vi "serial_read_write.vi"(10 "Enable Delayline":bool, 11 "VISA Refnum in":refnum<visa-resource-name>="COM4") -> ()   [LabVIEW 2024]
uses:
  <vilib>/Instr/_visa.llb/VISA Configure Serial Port (Instr).vi
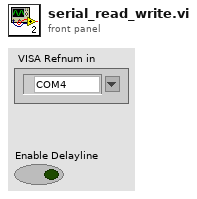
[diagram p1: front panel]
types:
  T1 = cluster{"baud rate":u32, "data bits":u16, "parity":dbl, "stop bits":u16, "flow control":u16}
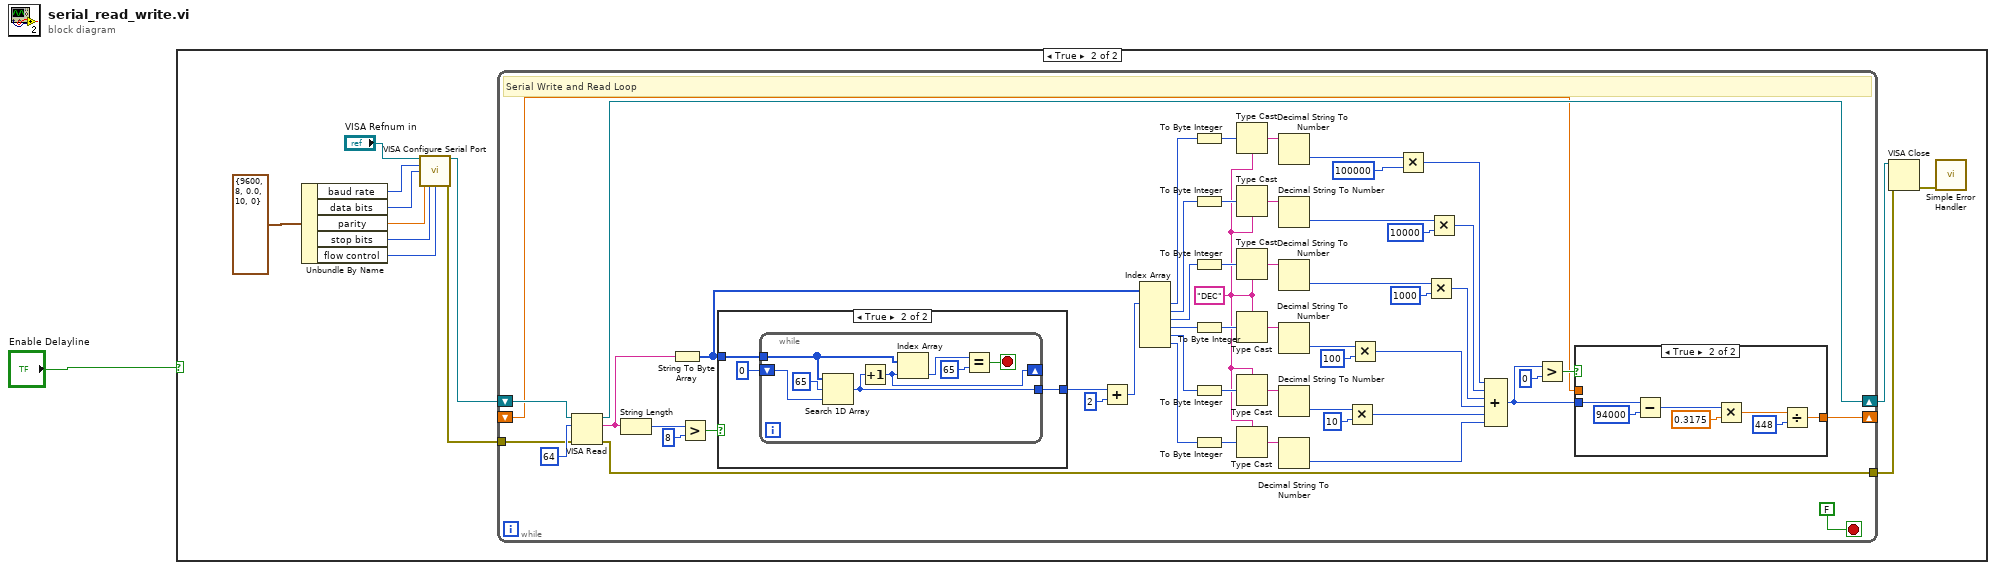
[diagram p0: block diagram]
diagram:
  n1 = case shown="True" "Enable Delayline" {
    frame False {
    }
    frame True {
      n2 = Unbundle By Name(T1 {"baud rate"=9600, "data bits"=8, "parity"=0.0, "stop bits"=10, "flow control"=0} ("Serial Settings")) -> ("baud rate"=w9:u32, "data bits"=w10:u16, "parity"=w11:dbl, "stop bits"=w12:u16, "flow control"=w4:u16)
      n3 = call-poly "VISA Configure Serial Port"("VISA resource name"="VISA Refnum in", "baud rate (9600)"=w9, "data bits (8)"=w10, "parity (0:none)"=w11, "stop bits (10: 1 bit)"=w12, "flow control (0:none)"=w4) -> ("VISA resource name out"=w2:refnum<visa-resource-name>, "error out"=w3:errorcluster)  [unwired: 4 in, 4 out]
      n4 = while {
        shift-right: [w66] -> w5
        shift-left: w2 -> [w32]
        tunnel: [w65] -> w6
        tunnel: w3 -> [w33]
        shift-right: [w15] -> _
        shift-left: _ -> [w14]
        stop <- FALSE stop-if-true
        w25 = "DEC"
        # "Serial Write and Read Loop"
        n5 = VISA Read(VISA resource name=w32, byte count=u32 64 ("Read Count"), error in (no error)=w33) -> (VISA resource name out=w66:refnum<visa-resource-name>, read buffer=w37:string, error out=w65:errorcluster)  [unwired: 1 out]
        n6 = String Length(string=w37) -> (length=w36:i32)
        n7 = String To Byte Array(string=w37) -> (unsigned byte array=w62:u8[])
        n8 = Greater?(x=w36, y=8) -> (0:w34:bool)
        n9 = case shown="True" w34 {
          tunnel: w62 -> [_ w78]
          tunnel: [_ w77] -> w60
          frame False {
          }
          frame True {
            n10 = while {
              shift-right: [w80] -> _
              shift-left: 0 -> [w82]
              tunnel: w78 -> [w83]
              tunnel: [w79] -> w77
              stop <- w81 stop-if-true
              n11 = Search 1D Array(1D array=w83, element=65, start index (0)=w82) -> (index of element=w79:i32)
              n12 = Increment(x=w79) -> (x+1=w80:i32)
              n13 = Index Array(array=w83, index=w80) -> (element=w85:u8)
              n14 = Equal?(x=w85, y=65) -> (x = y?=w81:bool)
            }
          }
        }
        n15 = Add(x=w60, y=2) -> (x+y=w61:i32)
        n16 = Index Array(array=w62, index #1=w61) -> (element #1=w59:u8, element #2=w58:u8, element #3=w57:u8, element #4=w56:u8, element #5=w55:u8, element #6=w27:u8)  [unwired: 5 in]
        n17 = To Byte Integer(number=w59) -> (8bit integer=w31:i8)
        n18 = To Byte Integer(number=w58) -> (8bit integer=w54:i8)
        n19 = To Byte Integer(number=w57) -> (8bit integer=w53:i8)
        n20 = To Byte Integer(number=w56) -> (8bit integer=w52:i8)
        n21 = To Byte Integer(number=w55) -> (8bit integer=w51:i8)
        n22 = To Byte Integer(number=w27) -> (8bit integer=w26:i8)
        n23 = Type Cast(type=w25, x=w31) -> (*(type *) &x=w30:string)
        n24 = Type Cast(type=w25, x=w54) -> (*(type *) &x=w50:string)
        n25 = Type Cast(type=w25, x=w53) -> (*(type *) &x=w49:string)
        n26 = Type Cast(type=w25, x=w52) -> (*(type *) &x=w48:string)
        n27 = Type Cast(type=w25, x=w51) -> (*(type *) &x=w47:string)
        n28 = Type Cast(type=w25, x=w26) -> (*(type *) &x=w20:string)
        n29 = Decimal String To Number(string=w30) -> (number=w23:i32)  [unwired: 2 in, 1 out]
        n30 = Decimal String To Number(string=w50) -> (number=w45:i32)  [unwired: 2 in, 1 out]
        n31 = Decimal String To Number(string=w49) -> (number=w44:i32)  [unwired: 2 in, 1 out]
        n32 = Decimal String To Number(string=w48) -> (number=w42:i32)  [unwired: 2 in, 1 out]
        n33 = Decimal String To Number(string=w47) -> (number=w22:i32)  [unwired: 2 in, 1 out]
        n34 = Decimal String To Number(string=w20) -> (number=w19:i32)  [unwired: 2 in, 1 out]
        n35 = Multiply(x=w22, y=10) -> (x*y=w24:i32)
        n36 = Multiply(x=w42, y=100) -> (x*y=w38:i32)
        n37 = Multiply(x=w23, y=100000) -> (x*y=w28:i32)
        n38 = Multiply(x=w44, y=1000) -> (x*y=w39:i32)
        n39 = Multiply(x=w45, y=10000) -> (x*y=w40:i32)
        n40 = Compound Arithmetic op=ADD(w28, w40, w39, w38, w24, w19) -> (w16:i32)
        n41 = Greater?(x=w16, y=0) -> (0:w17:bool)
        n42 = case shown="True" w17 {
          tunnel: [w68 w69] -> w15
          tunnel: w16 -> [_ w75]
          tunnel: w14 -> [w68 _]
          frame False {
          }
          frame True {
            n43 = Subtract(x=w75, y=94000) -> (x-y=w73:i32)
            n44 = Multiply(x=w73, y=0.3175) -> (x*y=w71:dbl)
            n45 = Divide(x=w71, y=448) -> (x/y=w69:dbl)
          }
        }
      }
      n46 = VISA Close(VISA resource name=w5, error in (no error)=w6) -> (error out=w7:errorcluster)
      n47 = call <vilib>:"Simple Error Handler.vi"("error in (no error)"=w7) -> ()  [unwired: 1 in, 8 out]
    }
  }
